vi "Collector.vi"(8 "error in":errorcluster) -> (0 "error out":errorcluster)   [LabVIEW 2015]
uses:
  Sprocket/src/Refname/Actuators.ctl
  Sprocket/src/Refname/Queues.ctl
  Sprocket/src/Action/Action Name.ctl
  Sprocket/src/Refname/Refname to String (Queue).vi
  Sprocket/lib/Sprocket.lvlib
panel:
  in  "intake power":dbl=0.5 format="%#_13g"
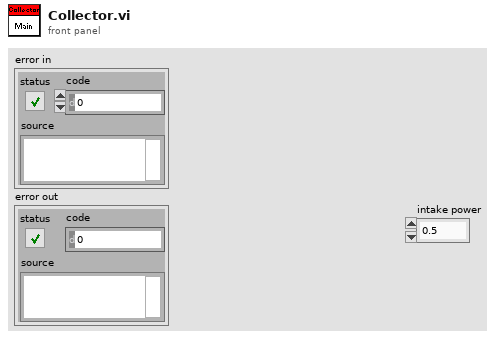
[diagram p1: front panel]
types:
  T1 = typedef "Sprocket.lvlib/Queues.ctl" = enum16{"Input", "Drive", "Collector", "Shifter", "Wedge"}
  T2 = typedef "Sprocket.lvlib/Actuators.ctl" = enum16{"Drive Motor 1 (R)", "Drive Motor 2 (R)", "Drive Motor 3 (R)", "Drive Motor 4 (L)", "Drive Motor 5 (L)", "Drive Motor 6 (L)", "Collector Motor", "Collector Solenoid", "Compressor", "SonicShifter", "Gyro", "UltraSonic Front Left", "UltraSonic Back Left", "Wedge Motor", "Wedge LS"}
  T3 = typedef "WPI_SolenoidDevRef.ctl" = cluster{"DevStatus":errorcluster, "Pneumatics Control Module":u8, "Forward Solenoid Channel":T4, "Reverse Solenoid Channel":T4}
  T4 = typedef "WPI_SolenoidChannel.ctl" = enum8{"Solenoid 0", "Solenoid 1", "Solenoid 2", "Solenoid 3", "Solenoid 4", "Solenoid 5", "Solenoid 6", "Solenoid 7", "Invalid"}
  T5 = typedef "WPI_MotorControlDeviceRef.ctl" = cluster{"DeviceStatus":errorcluster, "Type":T6, "PWM":cluster{"PWM Channel":T7, "DeadBand":T8}, "CAN":cluster{"Device Number":u8, "Control Mode":T9, "Semaphore":T10, "Max Vout":dbl, "TalonSRX Control Mode":T11}, "Invert":bool}
  T6 = typedef "WPI_MotorControlType.ctl" = enum16{"PWM", "CAN", "CANTalonSRX"}
  T7 = typedef "FPGA_DIOPWMChannel.ctl" = enum8{"PWM 0", "PWM 1", "PWM 2", "PWM 3", "PWM 4", "PWM 5", "PWM 6", "PWM 7", "PWM 8", "PWM 9", "PWM MXP 0", "PWM MXP 1", "PWM MXP 2", "PWM MXP 3", "PWM MXP 4", "PWM MXP 5", "PWM MXP 6", "PWM MXP 7", "PWM MXP 8", "PWM MXP 9", "Invalid"}
  T8 = typedef "WPI_PWMDeadband.ctl" = cluster{"Name":string, "maxPositivePwm":i32, "minPositivePwm":i32, "centerPwm":i32, "maxNegativePwm":i32, "minNegativePwm":i32, "angularRange":u16}
  T9 = typedef "WPI_CANJaguar_ControlMode.ctl" = enum8{"Percent VBus", "Current", "Speed", "Position", "Voltage"}
  T10 = typedef "Semaphore RefNum" = refnum<k1>
  T11 = typedef "WPI_CANTalonSRX_APIControlMode.ctl" = enum8{"Percent VBus", "Speed", "Position", "Slave", "Unchanged / Invalid", "Voltage Compensation", "Current", "Motion Profile"}
  T12 = typedef "Sprocket.lvlib/Action Name.ctl" = enum16{"No Action", "Drive Train Both", "Drive Train Rotate", "Drive Train Throttle", "Collector Motor Roll", "Collector Motor Eject", "Collector Motor Collect", "Collector Motor Stop", "Collector Extend", "Collector Retract", "Shifter High", "Shifter Low", "Collector Motor Stall", "Wedge Roll"}
  T13 = typedef "Sprocket.lvlib/Action.ctl" = cluster{"Name":T12, "Priority":i32, "Data":variant}
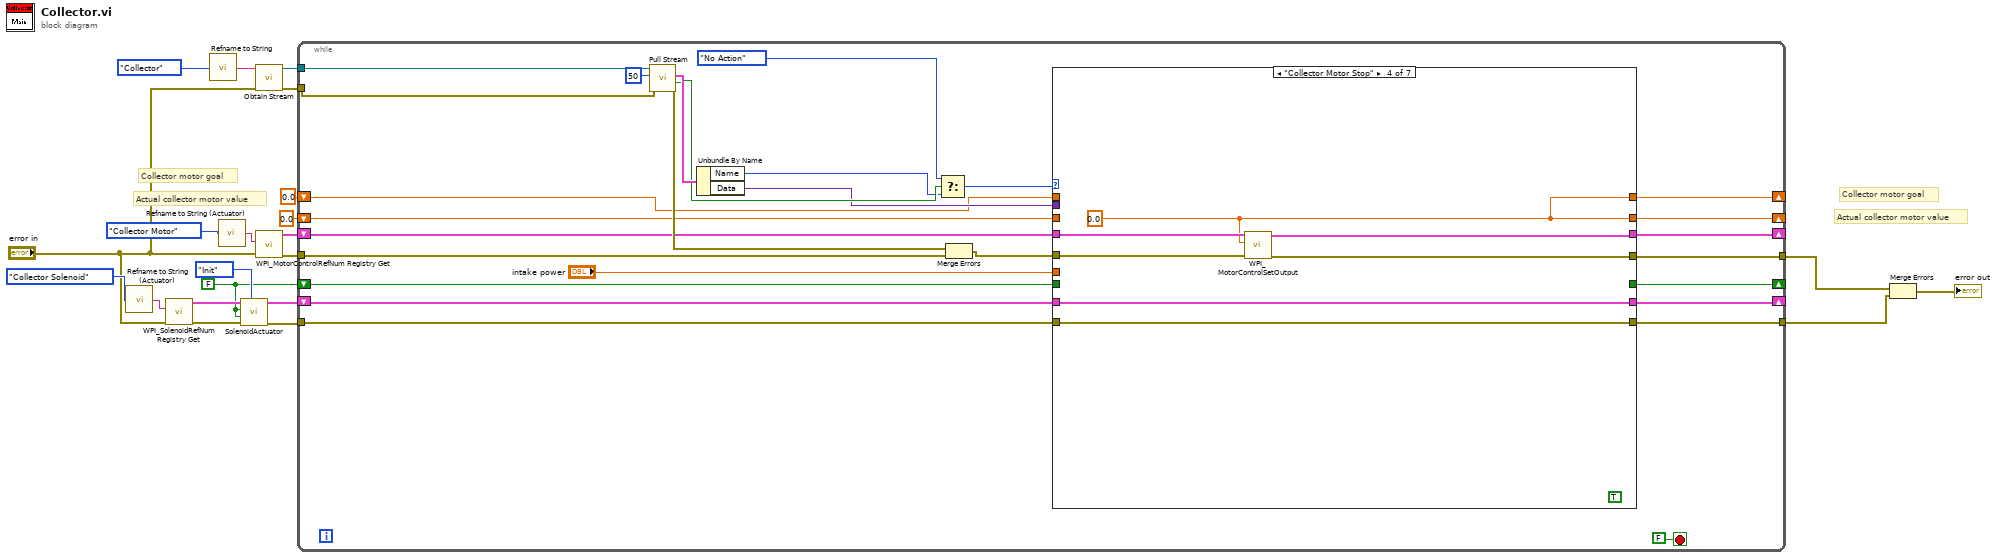
[diagram p0: block diagram]
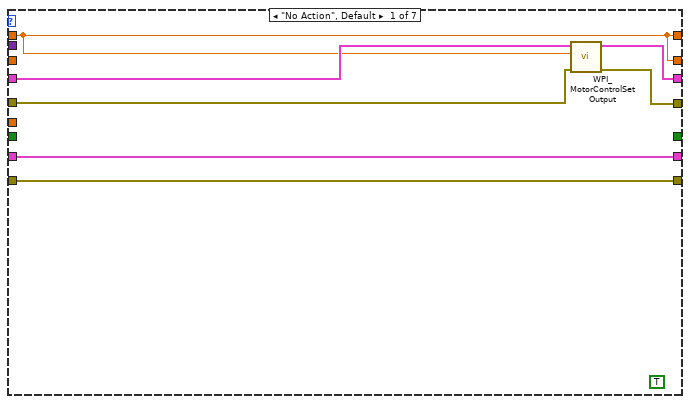
[diagram p2: hidden frame]
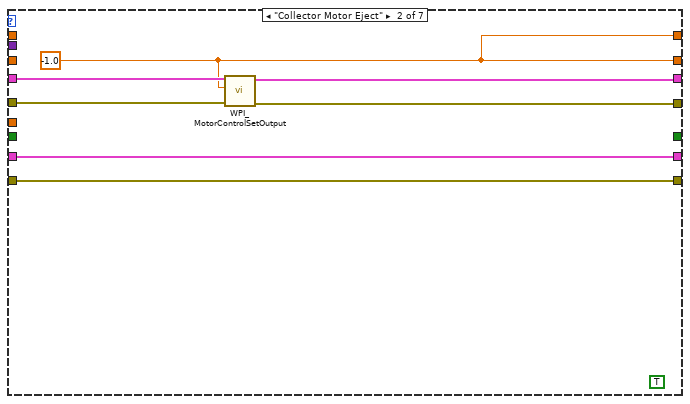
[diagram p3: hidden frame]
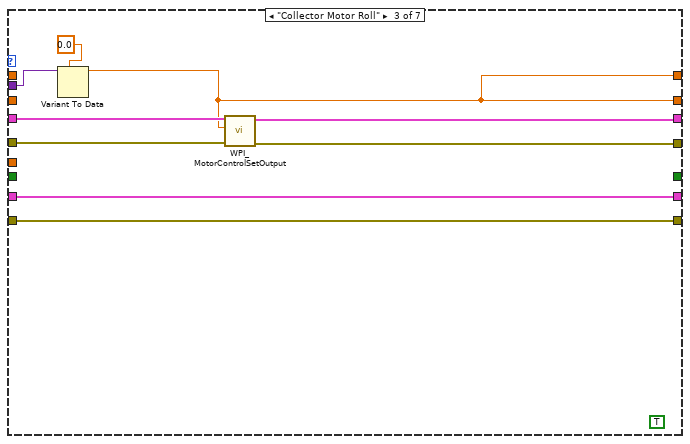
[diagram p4: hidden frame]
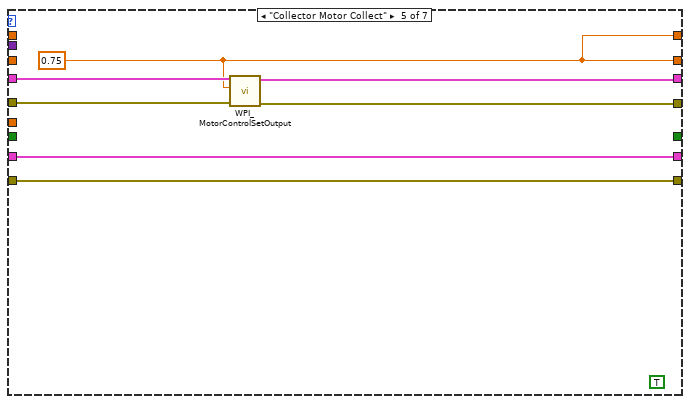
[diagram p5: hidden frame]
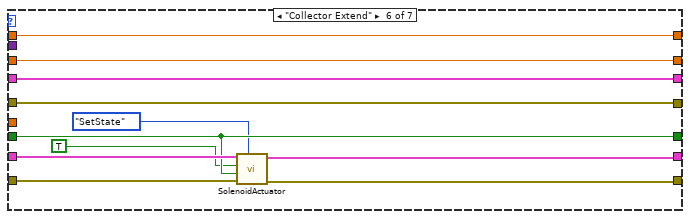
[diagram p6: hidden frame]
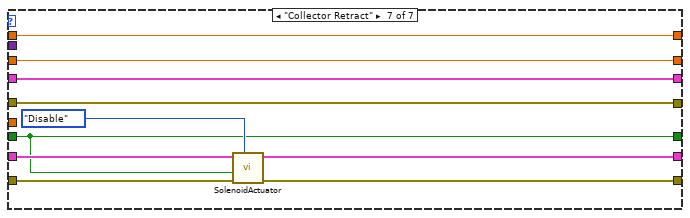
[diagram p7: hidden frame]
diagram:
  w4 = FALSE
  # "Collector motor goal"
  # "Actual collector motor value"
  # "Collector motor goal"
  # "Actual collector motor value"
  n1 = call "Refname to String (Actuator).vi"("Actuator Refname"=Actuators."Collector Solenoid") -> ("Refnum Name"=w14:string)
  n2 = call <vilib>:"WPI_SolenoidRefNum Registry Get.vi"("error in (no error)"="error in", "refnum name"=w14) -> ("error out"=w8:errorcluster, "SolenoidDevRef"=w5:T3)  [unwired: 8 in]
  n3 = call-poly "Refname to String.vi"("Queue Refname"=Queues."Collector" ("Refname (Queue)")) -> ("Refnum Name"=w1:string)
  n4 = call "Refname to String (Actuator).vi"("Actuator Refname"=Actuators."Collector Motor") -> ("Refnum Name"=w21:string)
  n5 = call "SolenoidActuator.vi"("Action"=enum16{"Init", "SetState", "Disable"}."Init", "error in"=w8, "Reverse Actuation"=w4, "Actuate?"=w4, "SolenoidDevRef"=w5) -> ("error out"=w7:errorcluster, "SolenoidDevRef out"=w6:T3)  [unwired: 5 in]
  n6 = call "Obtain Stream.vi"("error in (no error)"="error in", "Name"=w1) -> ("error out"=w19:errorcluster, "stream out"=w20:refnum<queue>)  [unwired: 8 in]
  n7 = call <vilib>:"WPI_MotorControlRefNum Registry Get.vi"("error in (no error)"="error in", "refnum name"=w21) -> ("error out"=w18:errorcluster, "MotorControlDevRef"=w17:T5)  [unwired: 8 in]
  n8 = while {
    tunnel: w20 -> [w24]
    tunnel: w19 -> [w31]
    tunnel: w18 -> [w38]
    shift-right: [w43] -> _
    shift-left: 0.0 -> [w27]
    shift-right: [w42] -> _
    shift-left: w17 -> [w29]
    tunnel: [w41] -> w12
    tunnel: w7 -> [w30]
    shift-right: [w37] -> _
    shift-left: w6 -> [w35]
    tunnel: [w36] -> w11
    shift-right: [w33] -> _
    shift-left: w4 -> [w34]
    shift-right: [w32] -> _
    shift-left: 0.0 -> [w28]
    stop <- FALSE stop-if-true
    n9 = call "Pull Stream.vi"("error in (no error)"=w31, "timeout in ms (-1)"=50, "stream in"=w24) -> ("error out"=w39:errorcluster, "timed out?"=w47:bool, "element"=w48:T13)  [unwired: 5 in, 1 out]
    n10 = Unbundle By Name(w48) -> ("Name"=w45:T12, "Data"=w44:variant)
    n11 = Select(t=Action_Name."No Action" ("Name"), s=w47, f=w45) -> (s? t:f=w25:T12)
    n12 = Merge Errors(w39, w38) -> (w40:errorcluster)
    n13 = case shown="\"Collector Motor Stop\"" w25 {
      tunnel: w44 -> [_ _ w65 _ _ _ _]
      tunnel: w40 -> [w55 w62 w71 w79 w86 w88 w107]
      tunnel: w29 -> [w56 w63 w72 w77 w84 w97 w106]
      tunnel: w27 -> [_ _ _ _ _ w96 w105]
      tunnel: [w50 w57 w64 w73 w80 w96 w105] -> w43
      tunnel: [w54 w61 w70 w78 w85 w88 w107] -> w41
      tunnel: [w53 w60 w69 w76 w83 w97 w106] -> w42
      tunnel: w35 -> [w52 w59 w68 w75 w82 w95 w104]
      tunnel: [w52 w59 w68 w75 w82 w92 w103] -> w37
      tunnel: w30 -> [w51 w58 w67 w74 w81 w94 w102]
      tunnel: [w51 w58 w67 w74 w81 w93 w101] -> w36
      tunnel: w34 -> [_ _ _ _ _ w91 w99]
      tunnel: [_ _ _ _ _ w91 w99] -> w33
      tunnel: [w50 w57 w64 w73 w80 w89 w98] -> w32
      tunnel: w28 -> [w50 _ _ _ _ w89 w98]
      tunnel: "intake power" -> [_ _ _ _ _ _ _]
      frame "No Action", Default {
        (unwired) TRUE
        n14 = call <vilib>:"WPI_MotorControlSetOutput.vi"("error in (no error)"=w55, "Output"=w50, "MotorControlDevRef"=w56) -> ("error out"=w54:errorcluster, "MotorControlDevRef"=w53:T5)  [unwired: 6 in, 1 out]
      }
      frame "Collector Motor Eject" {
        (unwired) TRUE
        w57 = -1.0
        n15 = call <vilib>:"WPI_MotorControlSetOutput.vi"("error in (no error)"=w62, "Output"=w57, "MotorControlDevRef"=w63) -> ("error out"=w61:errorcluster, "MotorControlDevRef"=w60:T5)  [unwired: 6 in, 1 out]
      }
      frame "Collector Motor Roll" {
        (unwired) TRUE
        n16 = Variant To Data(type=0.0, Variant=w65) -> (data=w64:dbl)  [unwired: 1 in, 1 out]
        n17 = call <vilib>:"WPI_MotorControlSetOutput.vi"("error in (no error)"=w71, "Output"=w64, "MotorControlDevRef"=w72) -> ("error out"=w70:errorcluster, "MotorControlDevRef"=w69:T5)  [unwired: 6 in, 1 out]
      }
      frame "Collector Motor Stop" {
        (unwired) TRUE
        w73 = 0.0
        n18 = call <vilib>:"WPI_MotorControlSetOutput.vi"("error in (no error)"=w79, "Output"=w73, "MotorControlDevRef"=w77) -> ("error out"=w78:errorcluster, "MotorControlDevRef"=w76:T5)  [unwired: 6 in, 1 out]
      }
      frame "Collector Motor Collect" {
        (unwired) TRUE
        w80 = 0.75
        n19 = call <vilib>:"WPI_MotorControlSetOutput.vi"("error in (no error)"=w86, "Output"=w80, "MotorControlDevRef"=w84) -> ("error out"=w85:errorcluster, "MotorControlDevRef"=w83:T5)  [unwired: 6 in, 1 out]
      }
      frame "Collector Extend" {
        n20 = call "SolenoidActuator.vi"("Action"=enum16{"Init", "SetState", "Disable"}."SetState", "error in"=w94, "Reverse Actuation"=w91, "Actuate?"=TRUE, "SolenoidDevRef"=w95) -> ("error out"=w93:errorcluster, "SolenoidDevRef out"=w92:T3)  [unwired: 5 in]
      }
      frame "Collector Retract" {
        n21 = call "SolenoidActuator.vi"("Action"=enum16{"Init", "SetState", "Disable"}."Disable", "error in"=w102, "Reverse Actuation"=w99, "SolenoidDevRef"=w104) -> ("error out"=w101:errorcluster, "SolenoidDevRef out"=w103:T3)  [unwired: 6 in]
      }
    }
  }
  n22 = Merge Errors(w12, w11) -> (→"error out":errorcluster)
